vi "Write batch mode.vi"(8 "error in (no error)":errorcluster, 10 "batch mode?":bool=TRUE, 11 "PuTTY Client in":refnum<class "PuTTY Client.lvclass">) -> (0 "error out":errorcluster, 3 "PuTTY Client out":refnum<class "PuTTY Client.lvclass">)   [LabVIEW 2020, in "NI_SSH.lvlib" / "PuTTY Client.lvclass"]
uses:
  <vilib>/net/SSH/Client/PuTTY/PuTTY Client.lvclass
  <vilib>/Utility/error.llb/Error Cluster From Error Code.vi
  <vilib>/ErrorRing/Error Ring.xnode
  <vilib>/net/SSH/Client/Generic/Generic Client.lvclass
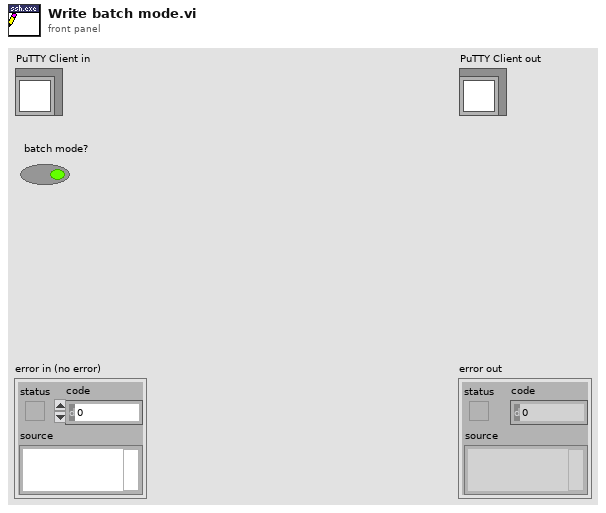
[diagram p1: front panel]
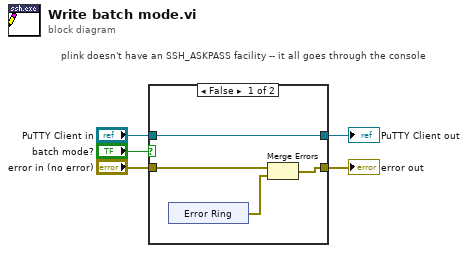
[diagram p0: block diagram]
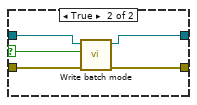
[diagram p2: hidden frame]
diagram:
  # "plink doesn't have an SSH_ASKPASS facility -- it all goes through the console"
  n1 = case shown="False" "batch mode?" {
    selector: "batch mode?" -> [_ w14]
    tunnel: [w6 w18] -> w5
    tunnel: [w9 w17] -> w4
    tunnel: "error in (no error)" -> [w7 w16]
    tunnel: "PuTTY Client in" -> [w9 w15]
    frame False {
      n2 = xnode ("Error Ring")() -> ("error out"=w8:errorcluster)
      n3 = Merge Errors(w7, w8) -> (w6:errorcluster)
    }
    frame True {
      n4 = call-parent "Write batch mode.vi"("error in (no error)"=w16, "batch mode?"=w14, "Generic Client in"=w15) -> ("error out"=w18:errorcluster, "Generic Client out"=w17:refnum<class "PuTTY Client.lvclass">)  [unwired: 7 in]
    }
  }
  "error out" <- w5
  "PuTTY Client out" <- w4
